vi "UMLEditor IsALLBFile.vi"(1 "path":path) -> (0 "path to VI library?":bool)   [LabVIEW 2014]
doc: "Decides by looking at the extension of a file name whether it is a VI library or directory. The purpose of this VI is to determine whether a non-existing parent path is meant to be a directory or VI library, so it doesn't try to look at file type or contents."
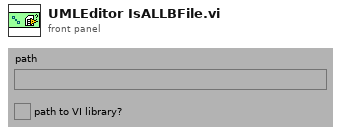
[diagram p1: front panel]
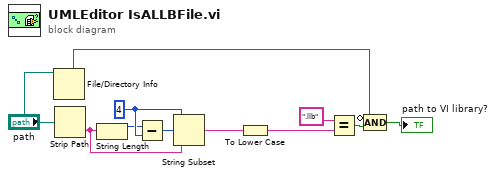
[diagram p0: block diagram]
diagram:
  w9 = 4
  n1 = File/Directory Info(path="path") -> (directory=w1:bool)  [unwired: 1 in, 6 out]
  n2 = Strip Path(path="path") -> (name=w11:string)  [unwired: 1 out]
  n3 = String Length(string=w11) -> (length=w8:i32)
  n4 = Subtract(x=w8, y=w9) -> (x-y=w10:i32)
  n5 = String Subset(string=w11, offset (0)=w10, length (rest)=w9) -> (substring=w7:string)
  n6 = To Lower Case(string=w7) -> (all lower case string=w6:string)
  n7 = Equal?(x=".llb", y=w6) -> (x = y?=w4:bool)
  n8 = Compound Arithmetic op=AND(invert w1, w4) -> (→"path to VI library?":bool)
